vi "Lab Panel V4.90.vi"() -> ()   [LabVIEW 2013] (continued)
                            n1480 = local write "RESULT LAB05-2"(TRUE) -> ()
                            n1481 = local write "DISP LAB05-2"(w2794) -> ()
                          }
                        }
                      }
                      frame False {
                      }
                    }
                  }
                }
              }
            }
          }
          frame #6 {
            # "end test & close test files"
            n1482 = local read "MAIL SETTINGS"() -> (w2800:T7)
            n1483 = Unbundle(w2800) -> ("OUT SERVER ADDRESS"=w2799:string, "FROM ACCOUNT"=w2798:string)  [unwired: 5 out]
            n1484 = stacked-sequence {
              tunnel: w2810 -> [_ _ _ _ _ _ _ _ _ _]
              tunnel: w2811 -> [_ _ _ _ _ _ _ _ _ _]
              tunnel: w2809 -> [_ _ _ _ _ _ _ _ _ _]
              tunnel: w2808 -> [_ _ _ _ _ _ _ _ _ _]
              tunnel: w2807 -> [_ _ _ _ _ _ _ _ _ _]
              tunnel: w2806 -> [_ _ _ _ _ _ _ _ _ _]
              tunnel: w2805 -> [_ _ _ _ _ _ _ _ _ _]
              tunnel: w2804 -> [_ _ _ _ _ _ _ _ _ _]
              tunnel: w2803 -> [_ _ _ _ _ _ _ _ _ _]
              tunnel: w2802 -> [_ _ _ _ _ _ _ _ _ _]
              tunnel: w2799 -> [w2815 w2867 w2915 w2962 w3009 w3056 w3103 w3150 w3197 w3244]
              tunnel: w2798 -> [w2814 w2866 w2914 w2961 w3008 w3055 w3102 w3149 w3196 w3243]
              tunnel: "Mail Test File To:" -> [w2813 w2865 w2913 w2960 w3007 w3054 w3101 w3148 w3195 w3242]
              tunnel: "Mail Test Fail" -> [w2812 w2864 w2912 w2959 w3006 w3053 w3100 w3147 w3194 w3241]
              frame #0 {
                # "LAB01-1"
                n1485 = local read "DISP LAB01-1"() -> (w2819:T4)
                n1486 = local read "run lab01-1"() -> (w2816:bool)
                n1487 = local read "TDMS LAB01-1"() -> (w2817:refnum<k34>)
                n1488 = Unbundle(w2819) -> ("CYCLE"=w2820:dbl, "STATUS"=w2818:string)  [unwired: 1 out]
                n1489 = case shown="True" w2816 {
                  tunnel: w2820 -> [_ w2826]
                  tunnel: w2819 -> [_ w2828]
                  tunnel: w2818 -> [_ w2825]
                  tunnel: w2817 -> [_ w2827]
                  tunnel: w2815 -> [_ w2824]
                  tunnel: w2814 -> [_ w2823]
                  tunnel: w2813 -> [_ w2822]
                  tunnel: w2812 -> [_ w2821]
                  frame False {
                  }
                  frame True {
                    n1490 = Not Equal?(x=w2825, y="RUN") -> (x != y?=w2829:bool)
                    n1491 = Greater?(x=w2826, y=2.0) -> (0:w2831:bool)
                    n1492 = And(x=w2831, y=w2829) -> (x .and. y?=w2830:bool)
                    n1493 = case shown="True" w2830 {
                      tunnel: w2828 -> [_ w2841]
                      tunnel: w2827 -> [_ w2840]
                      tunnel: w2826 -> [_ w2839]
                      tunnel: w2825 -> [_ w2838]
                      tunnel: w2824 -> [_ w2837]
                      tunnel: w2823 -> [_ w2836]
                      tunnel: w2822 -> [_ w2835]
                      tunnel: w2821 -> [_ w2834]
                      frame False {
                      }
                      frame True {
                        n1494 = stacked-sequence {
                          tunnel: w2841 -> [w2845 _ _]
                          tunnel: w2840 -> [_ w2847 _]
                          tunnel: w2839 -> [_ _ _]
                          tunnel: w2838 -> [_ _ w2853]
                          tunnel: w2837 -> [_ _ w2852]
                          tunnel: w2836 -> [_ _ w2851]
                          tunnel: w2835 -> [_ _ w2850]
                          tunnel: w2834 -> [_ _ w2849]
                          frame #0 {
                            w2842 = FALSE
                            n1495 = local write "mail control"("END") -> ()
                            n1496 = Bundle(cluster=w2845) -> (w2844:T4)  [unwired: 3 in]
                            n1497 = local write "DISP LAB01-1"(w2844) -> ()
                            n1498 = local write "O/I  LAB01-1"(w2842) -> ()
                            n1499 = local write "run lab01-1"(w2842) -> ()
                            n1500 = local write "RUN LAB01-1"(w2842) -> ()
                          }
                          frame #1 {
                            n1501 = TDMS Close(11:w2847) -> (0:w2846:errorcluster)  [unwired: 1 in, 1 out]
                            n1502 = local write "data file error"(w2846) -> ()
                          }
                          frame #2 {
                            n1503 = stacked-sequence {
                              tunnel: "LAB01-1" -> [w2855 w2857 _]
                              tunnel: w2853 -> [_ w2863 _]
                              tunnel: w2852 -> [_ w2862 _]
                              tunnel: w2851 -> [_ w2861 _]
                              tunnel: w2850 -> [_ w2860 _]
                              tunnel: w2849 -> [_ w2859 _]
                              frame #0 {
                                n1504 = call "sub vi - defrag tdms v1.vi"("panel id"=w2855) -> ("error out"=w2854:errorcluster)  [unwired: 10 in]
                                n1505 = local write "data file error"(w2854) -> ()
                              }
                              frame #1 {
                                n1506 = Bundle("STATUS"=w2863, "OUT SERVER ADDRESS"=w2862, "FROM ACCOUNT"=w2861, "Mail Test File To:"=w2860, "Mail Test Fail"=w2859) -> (w2856:T25)  [unwired: 1 in]
                                n1507 = call "Save data file (pass-fail) v5.vi"("Input Cluster"=w2856, "panel id"=w2857) -> ("network file save error"=w2858:errorcluster)  [unwired: 8 in, 1 out]
                                n1508 = local write "data file error"(w2858) -> ()
                              }
                              frame #2 {
                              }
                            }
                          }
                        }
                      }
                    }
                  }
                }
              }
              frame #1 {
                # "LAB01-2"
                n1509 = local read "run lab01-2"() -> (w2868:bool)
                n1510 = case shown="True" w2868 {
                  tunnel: w2867 -> [_ w2872]
                  tunnel: w2866 -> [_ w2871]
                  tunnel: w2865 -> [_ w2870]
                  tunnel: w2864 -> [_ w2869]
                  frame False {
                  }
                  frame True {
                    n1511 = local read "DISP LAB01-2"() -> (w2880:T4)
                    n1512 = local read "TDMS LAB01-2"() -> (w2879:refnum<k34>)
                    n1513 = Unbundle(w2880) -> ("CYCLE"=w2874:dbl, "STATUS"=w2873:string)  [unwired: 1 out]
                    n1514 = Not Equal?(x=w2873, y="RUN") -> (x != y?=w2876:bool)
                    n1515 = Greater?(x=w2874, y=2.0) -> (0:w2877:bool)
                    n1516 = And(x=w2877, y=w2876) -> (x .and. y?=w2875:bool)
                    n1517 = case shown="True" w2875 {
                      tunnel: w2880 -> [_ w2889]
                      tunnel: w2879 -> [_ w2888]
                      tunnel: w2874 -> [_ w2887]
                      tunnel: w2873 -> [_ w2886]
                      tunnel: w2872 -> [_ w2885]
                      tunnel: w2871 -> [_ w2884]
                      tunnel: w2870 -> [_ w2883]
                      tunnel: w2869 -> [_ w2882]
                      frame False {
                      }
                      frame True {
                        n1518 = stacked-sequence {
                          tunnel: w2889 -> [w2892 _ _]
                          tunnel: w2888 -> [_ w2894 _]
                          tunnel: w2887 -> [_ _ _]
                          tunnel: w2886 -> [_ _ w2900]
                          tunnel: w2885 -> [_ _ w2899]
                          tunnel: w2884 -> [_ _ w2898]
                          tunnel: w2883 -> [_ _ w2897]
                          tunnel: w2882 -> [_ _ w2896]
                          frame #0 {
                            w2890 = FALSE
                            n1519 = local write "mail control"("END") -> ()
                            n1520 = Bundle(cluster=w2892) -> (w2893:T4)  [unwired: 3 in]
                            n1521 = local write "RUN LAB01-2"(w2890) -> ()
                            n1522 = local write "run lab01-2"(w2890) -> ()
                            n1523 = local write "O/I  LAB01-2"(w2890) -> ()
                            n1524 = local write "DISP LAB01-2"(w2893) -> ()
                          }
                          frame #1 {
                            n1525 = TDMS Close(11:w2894) -> (0:w2895:errorcluster)  [unwired: 1 in, 1 out]
                            n1526 = local write "data file error"(w2895) -> ()
                          }
                          frame #2 {
                            n1527 = stacked-sequence {
                              tunnel: "LAB01-2" -> [w2903 w2904]
                              tunnel: w2900 -> [_ w2909]
                              tunnel: w2899 -> [_ w2908]
                              tunnel: w2898 -> [_ w2907]
                              tunnel: w2897 -> [_ w2906]
                              tunnel: w2896 -> [_ w2905]
                              frame #0 {
                                n1528 = call "sub vi - defrag tdms v1.vi"("panel id"=w2903) -> ("error out"=w2902:errorcluster)  [unwired: 10 in]
                                n1529 = local write "data file error"(w2902) -> ()
                              }
                              frame #1 {
                                n1530 = Bundle("STATUS"=w2909, "OUT SERVER ADDRESS"=w2908, "FROM ACCOUNT"=w2907, "Mail Test File To:"=w2906, "Mail Test Fail"=w2905) -> (w2911:T25)  [unwired: 1 in]
                                n1531 = call "Save data file (pass-fail) v5.vi"("Input Cluster"=w2911, "panel id"=w2904) -> ("network file save error"=w2910:errorcluster)  [unwired: 8 in, 1 out]
                                n1532 = local write "data file error"(w2910) -> ()
                              }
                            }
                          }
                        }
                      }
                    }
                  }
                }
              }
              frame #2 {
                # "LAB02-1"
                n1533 = local read "run lab02-1"() -> (w2916:bool)
                n1534 = case shown="True" w2916 {
                  tunnel: w2915 -> [_ w2920]
                  tunnel: w2914 -> [_ w2919]
                  tunnel: w2913 -> [_ w2918]
                  tunnel: w2912 -> [_ w2917]
                  frame False {
                  }
                  frame True {
                    n1535 = local read "DISP LAB02-1"() -> (w2928:T4)
                    n1536 = Unbundle(w2928) -> ("CYCLE"=w2924:dbl, "STATUS"=w2921:string)  [unwired: 1 out]
                    n1537 = local read "TDMS LAB02-1"() -> (w2927:refnum<k34>)
                    n1538 = Not Equal?(x=w2921, y="RUN") -> (x != y?=w2923:bool)
                    n1539 = Greater?(x=w2924, y=2.0) -> (0:w2925:bool)
                    n1540 = And(x=w2925, y=w2923) -> (x .and. y?=w2922:bool)
                    n1541 = case shown="True" w2922 {
                      tunnel: w2928 -> [_ w2936]
                      tunnel: w2927 -> [_ w2935]
                      tunnel: w2921 -> [_ w2934]
                      tunnel: w2920 -> [_ w2933]
                      tunnel: w2919 -> [_ w2932]
                      tunnel: w2918 -> [_ w2931]
                      tunnel: w2917 -> [_ w2930]
                      frame False {
                      }
                      frame True {
                        n1542 = stacked-sequence {
                          tunnel: w2936 -> [w2939 _ _]
                          tunnel: w2935 -> [_ w2941 _]
                          tunnel: w2934 -> [_ _ w2947]
                          tunnel: w2933 -> [_ _ w2946]
                          tunnel: w2932 -> [_ _ w2945]
                          tunnel: w2931 -> [_ _ w2944]
                          tunnel: w2930 -> [_ _ w2943]
                          frame #0 {
                            w2937 = FALSE
                            n1543 = local write "mail control"("END") -> ()
                            n1544 = Bundle(cluster=w2939) -> (w2940:T4)  [unwired: 3 in]
                            n1545 = local write "O/I  LAB02-1"(w2937) -> ()
                            n1546 = local write "RUN LAB02-1"(w2937) -> ()
                            n1547 = local write "run lab02-1"(w2937) -> ()
                            n1548 = local write "DISP LAB02-1"(w2940) -> ()
                          }
                          frame #1 {
                            n1549 = TDMS Close(11:w2941) -> (0:w2942:errorcluster)  [unwired: 1 in, 1 out]
                            n1550 = local write "data file error"(w2942) -> ()
                          }
                          frame #2 {
                            n1551 = stacked-sequence {
                              tunnel: "LAB02-1" -> [w2950 w2957]
                              tunnel: w2947 -> [_ w2955]
                              tunnel: w2946 -> [_ w2954]
                              tunnel: w2945 -> [_ w2953]
                              tunnel: w2944 -> [_ w2952]
                              tunnel: w2943 -> [_ w2951]
                              frame #0 {
                                n1552 = call "sub vi - defrag tdms v1.vi"("panel id"=w2950) -> ("error out"=w2949:errorcluster)  [unwired: 10 in]
                                n1553 = local write "data file error"(w2949) -> ()
                              }
                              frame #1 {
                                n1554 = Bundle("STATUS"=w2955, "OUT SERVER ADDRESS"=w2954, "FROM ACCOUNT"=w2953, "Mail Test File To:"=w2952, "Mail Test Fail"=w2951) -> (w2956:T25)  [unwired: 1 in]
                                n1555 = call "Save data file (pass-fail) v5.vi"("Input Cluster"=w2956, "panel id"=w2957) -> ("network file save error"=w2958:errorcluster)  [unwired: 8 in, 1 out]
                                n1556 = local write "data file error"(w2958) -> ()
                              }
                            }
                          }
                        }
                      }
                    }
                  }
                }
              }
              frame #3 {
                # "LAB02-2"
                n1557 = local read "run lab02-2"() -> (w2963:bool)
                n1558 = case shown="True" w2963 {
                  tunnel: w2962 -> [_ w2967]
                  tunnel: w2961 -> [_ w2966]
                  tunnel: w2960 -> [_ w2965]
                  tunnel: w2959 -> [_ w2964]
                  frame False {
                  }
                  frame True {
                    n1559 = local read "DISP LAB02-2"() -> (w2975:T4)
                    n1560 = local read "TDMS LAB02-2"() -> (w2974:refnum<k34>)
                    n1561 = Unbundle(w2975) -> ("CYCLE"=w2971:dbl, "STATUS"=w2968:string)  [unwired: 1 out]
                    n1562 = Not Equal?(x=w2968, y="RUN") -> (x != y?=w2970:bool)
                    n1563 = Greater?(x=w2971, y=2.0) -> (0:w2972:bool)
                    n1564 = And(x=w2972, y=w2970) -> (x .and. y?=w2969:bool)
                    n1565 = case shown="True" w2969 {
                      tunnel: w2975 -> [_ w2983]
                      tunnel: w2974 -> [_ w2982]
                      tunnel: w2968 -> [_ w2981]
                      tunnel: w2967 -> [_ w2980]
                      tunnel: w2966 -> [_ w2979]
                      tunnel: w2965 -> [_ w2978]
                      tunnel: w2964 -> [_ w2977]
                      frame False {
                      }
                      frame True {
                        n1566 = stacked-sequence {
                          tunnel: w2983 -> [w2986 _ _]
                          tunnel: w2982 -> [_ w2988 _]
                          tunnel: w2981 -> [_ _ w2994]
                          tunnel: w2980 -> [_ _ w2993]
                          tunnel: w2979 -> [_ _ w2992]
                          tunnel: w2978 -> [_ _ w2991]
                          tunnel: w2977 -> [_ _ w2990]
                          frame #0 {
                            w2984 = FALSE
                            n1567 = local write "mail control"("END") -> ()
                            n1568 = Bundle(cluster=w2986) -> (w2987:T4)  [unwired: 3 in]
                            n1569 = local write "O/I  LAB02-2"(w2984) -> ()
                            n1570 = local write "run lab02-2"(w2984) -> ()
                            n1571 = local write "RUN LAB02-2"(w2984) -> ()
                            n1572 = local write "DISP LAB02-2"(w2987) -> ()
                          }
                          frame #1 {
                            n1573 = TDMS Close(11:w2988) -> (0:w2989:errorcluster)  [unwired: 1 in, 1 out]
                            n1574 = local write "data file error"(w2989) -> ()
                          }
                          frame #2 {
                            n1575 = stacked-sequence {
                              tunnel: "LAB02-2" -> [w2997 w3003]
                              tunnel: w2994 -> [_ w3002]
                              tunnel: w2993 -> [_ w3001]
                              tunnel: w2992 -> [_ w3000]
                              tunnel: w2991 -> [_ w2999]
                              tunnel: w2990 -> [_ w2998]
                              frame #0 {
                                n1576 = call "sub vi - defrag tdms v1.vi"("panel id"=w2997) -> ("error out"=w2996:errorcluster)  [unwired: 10 in]
                                n1577 = local write "data file error"(w2996) -> ()
                              }
                              frame #1 {
                                n1578 = Bundle("STATUS"=w3002, "OUT SERVER ADDRESS"=w3001, "FROM ACCOUNT"=w3000, "Mail Test File To:"=w2999, "Mail Test Fail"=w2998) -> (w3005:T25)  [unwired: 1 in]
                                n1579 = call "Save data file (pass-fail) v5.vi"("Input Cluster"=w3005, "panel id"=w3003) -> ("network file save error"=w3004:errorcluster)  [unwired: 8 in, 1 out]
                                n1580 = local write "data file error"(w3004) -> ()
                              }
                            }
                          }
                        }
                      }
                    }
                  }
                }
              }
              frame #4 {
                # "LAB03-1"
                n1581 = local read "run lab03-1"() -> (w3010:bool)
                n1582 = case shown="True" w3010 {
                  tunnel: w3009 -> [_ w3014]
                  tunnel: w3008 -> [_ w3013]
                  tunnel: w3007 -> [_ w3012]
                  tunnel: w3006 -> [_ w3011]
                  frame False {
                  }
                  frame True {
                    n1583 = local read "DISP LAB03-1"() -> (w3022:T4)
                    n1584 = local read "TDMS LAB03-1"() -> (w3021:refnum<k34>)
                    n1585 = Unbundle(w3022) -> ("CYCLE"=w3018:dbl, "STATUS"=w3015:string)  [unwired: 1 out]
                    n1586 = Not Equal?(x=w3015, y="RUN") -> (x != y?=w3017:bool)
                    n1587 = Greater?(x=w3018, y=2.0) -> (0:w3019:bool)
                    n1588 = And(x=w3019, y=w3017) -> (x .and. y?=w3016:bool)
                    n1589 = case shown="True" w3016 {
                      tunnel: w3022 -> [_ w3030]
                      tunnel: w3021 -> [_ w3029]
                      tunnel: w3015 -> [_ w3028]
                      tunnel: w3014 -> [_ w3027]
                      tunnel: w3013 -> [_ w3026]
                      tunnel: w3012 -> [_ w3025]
                      tunnel: w3011 -> [_ w3024]
                      frame False {
                      }
                      frame True {
                        n1590 = stacked-sequence {
                          tunnel: w3030 -> [w3033 _ _]
                          tunnel: w3029 -> [_ w3035 _]
                          tunnel: w3028 -> [_ _ w3041]
                          tunnel: w3027 -> [_ _ w3040]
                          tunnel: w3026 -> [_ _ w3039]
                          tunnel: w3025 -> [_ _ w3038]
                          tunnel: w3024 -> [_ _ w3037]
                          frame #0 {
                            w3031 = FALSE
                            n1591 = local write "mail control"("END") -> ()
                            n1592 = Bundle(cluster=w3033) -> (w3034:T4)  [unwired: 3 in]
                            n1593 = local write "O/I  LAB03-1"(w3031) -> ()
                            n1594 = local write "run lab03-1"(w3031) -> ()
                            n1595 = local write "RUN LAB03-1"(w3031) -> ()
                            n1596 = local write "DISP LAB03-1"(w3034) -> ()
                          }
                          frame #1 {
                            n1597 = TDMS Close(11:w3035) -> (0:w3036:errorcluster)  [unwired: 1 in, 1 out]
                            n1598 = local write "data file error"(w3036) -> ()
                          }
                          frame #2 {
                            n1599 = stacked-sequence {
                              tunnel: "LAB03-1" -> [w3044 w3050]
                              tunnel: w3041 -> [_ w3049]
                              tunnel: w3040 -> [_ w3048]
                              tunnel: w3039 -> [_ w3047]
                              tunnel: w3038 -> [_ w3046]
                              tunnel: w3037 -> [_ w3045]
                              frame #0 {
                                n1600 = call "sub vi - defrag tdms v1.vi"("panel id"=w3044) -> ("error out"=w3043:errorcluster)  [unwired: 10 in]
                                n1601 = local write "data file error"(w3043) -> ()
                              }
                              frame #1 {
                                n1602 = Bundle("STATUS"=w3049, "OUT SERVER ADDRESS"=w3048, "FROM ACCOUNT"=w3047, "Mail Test File To:"=w3046, "Mail Test Fail"=w3045) -> (w3052:T25)  [unwired: 1 in]
                                n1603 = call "Save data file (pass-fail) v5.vi"("Input Cluster"=w3052, "panel id"=w3050) -> ("network file save error"=w3051:errorcluster)  [unwired: 8 in, 1 out]
                                n1604 = local write "data file error"(w3051) -> ()
                              }
                            }
                          }
                        }
                      }
                    }
                  }
                }
              }
              frame #5 {
                # "LAB03-2"
                n1605 = local read "run lab03-2"() -> (w3057:bool)
                n1606 = case shown="True" w3057 {
                  tunnel: w3056 -> [_ w3061]
                  tunnel: w3055 -> [_ w3060]
                  tunnel: w3054 -> [_ w3059]
                  tunnel: w3053 -> [_ w3058]
                  frame False {
                  }
                  frame True {
                    n1607 = local read "DISP LAB03-2"() -> (w3069:T4)
                    n1608 = Unbundle(w3069) -> ("CYCLE"=w3065:dbl, "STATUS"=w3062:string)  [unwired: 1 out]
                    n1609 = local read "TDMS LAB03-2"() -> (w3068:refnum<k34>)
                    n1610 = Not Equal?(x=w3062, y="RUN") -> (x != y?=w3064:bool)
                    n1611 = Greater?(x=w3065, y=2.0) -> (0:w3066:bool)
                    n1612 = And(x=w3066, y=w3064) -> (x .and. y?=w3063:bool)
                    n1613 = case shown="True" w3063 {
                      tunnel: w3069 -> [_ w3077]
                      tunnel: w3068 -> [_ w3076]
                      tunnel: w3062 -> [_ w3075]
                      tunnel: w3061 -> [_ w3074]
                      tunnel: w3060 -> [_ w3073]
                      tunnel: w3059 -> [_ w3072]
                      tunnel: w3058 -> [_ w3071]
                      frame False {
                      }
                      frame True {
                        n1614 = stacked-sequence {
                          tunnel: w3077 -> [w3080 _ _]
                          tunnel: w3076 -> [_ w3082 _]
                          tunnel: w3075 -> [_ _ w3088]
                          tunnel: w3074 -> [_ _ w3087]
                          tunnel: w3073 -> [_ _ w3086]
                          tunnel: w3072 -> [_ _ w3085]
                          tunnel: w3071 -> [_ _ w3084]
                          frame #0 {
                            w3078 = FALSE
                            n1615 = local write "mail control"("END") -> ()
                            n1616 = Bundle(cluster=w3080) -> (w3081:T4)  [unwired: 3 in]
                            n1617 = local write "RUN LAB03-2"(w3078) -> ()
                            n1618 = local write "O/I  LAB03-2"(w3078) -> ()
                            n1619 = local write "DISP LAB03-2"(w3081) -> ()
                            n1620 = local write "run lab03-2"(w3078) -> ()
                          }
                          frame #1 {
                            n1621 = TDMS Close(11:w3082) -> (0:w3083:errorcluster)  [unwired: 1 in, 1 out]
                            n1622 = local write "data file error"(w3083) -> ()
                          }
                          frame #2 {
                            n1623 = stacked-sequence {
                              tunnel: "LAB03-2" -> [w3091 w3092]
                              tunnel: w3088 -> [_ w3097]
                              tunnel: w3087 -> [_ w3096]
                              tunnel: w3086 -> [_ w3095]
                              tunnel: w3085 -> [_ w3094]
                              tunnel: w3084 -> [_ w3093]
                              frame #0 {
                                n1624 = call "sub vi - defrag tdms v1.vi"("panel id"=w3091) -> ("error out"=w3090:errorcluster)  [unwired: 10 in]
                                n1625 = local write "data file error"(w3090) -> ()
                              }
                              frame #1 {
                                n1626 = Bundle("STATUS"=w3097, "OUT SERVER ADDRESS"=w3096, "FROM ACCOUNT"=w3095, "Mail Test File To:"=w3094, "Mail Test Fail"=w3093) -> (w3099:T25)  [unwired: 1 in]
                                n1627 = call "Save data file (pass-fail) v5.vi"("Input Cluster"=w3099, "panel id"=w3092) -> ("network file save error"=w3098:errorcluster)  [unwired: 8 in, 1 out]
                                n1628 = local write "data file error"(w3098) -> ()
                              }
                            }
                          }
                        }
                      }
                    }
                  }
                }
              }
              frame #6 {
                # "LAB04-1"
                n1629 = local read "run lab04-1"() -> (w3104:bool)
                n1630 = case shown="True" w3104 {
                  tunnel: w3103 -> [_ w3108]
                  tunnel: w3102 -> [_ w3107]
                  tunnel: w3101 -> [_ w3106]
                  tunnel: w3100 -> [_ w3105]
                  frame False {
                  }
                  frame True {
                    n1631 = local read "DISP LAB04-1"() -> (w3116:T4)
                    n1632 = Unbundle(w3116) -> ("CYCLE"=w3112:dbl, "STATUS"=w3109:string)  [unwired: 1 out]
                    n1633 = local read "TDMS LAB04-1"() -> (w3115:refnum<k34>)
                    n1634 = Not Equal?(x=w3109, y="RUN") -> (x != y?=w3111:bool)
                    n1635 = Greater?(x=w3112, y=2.0) -> (0:w3113:bool)
                    n1636 = And(x=w3113, y=w3111) -> (x .and. y?=w3110:bool)
                    n1637 = case shown="True" w3110 {
                      tunnel: w3116 -> [_ w3124]
                      tunnel: w3115 -> [_ w3123]
                      tunnel: w3109 -> [_ w3122]
                      tunnel: w3108 -> [_ w3121]
                      tunnel: w3107 -> [_ w3120]
                      tunnel: w3106 -> [_ w3119]
                      tunnel: w3105 -> [_ w3118]
                      frame False {
                      }
                      frame True {
                        n1638 = stacked-sequence {
                          tunnel: w3124 -> [w3127 _ _]
                          tunnel: w3123 -> [_ w3129 _]
                          tunnel: w3122 -> [_ _ w3135]
                          tunnel: w3121 -> [_ _ w3134]
                          tunnel: w3120 -> [_ _ w3133]
                          tunnel: w3119 -> [_ _ w3132]
                          tunnel: w3118 -> [_ _ w3131]
                          frame #0 {
                            w3125 = FALSE
                            n1639 = local write "mail control"("END") -> ()
                            n1640 = Bundle(cluster=w3127) -> (w3128:T4)  [unwired: 3 in]
                            n1641 = local write "RUN LAB04-1"(w3125) -> ()
                            n1642 = local write "O/I  LAB04-1"(w3125) -> ()
                            n1643 = local write "run lab04-1"(w3125) -> ()
                            n1644 = local write "DISP LAB04-1"(w3128) -> ()
                          }
                          frame #1 {
                            n1645 = TDMS Close(11:w3129) -> (0:w3130:errorcluster)  [unwired: 1 in, 1 out]
                            n1646 = local write "data file error"(w3130) -> ()
                          }
                          frame #2 {
                            n1647 = stacked-sequence {
                              tunnel: "LAB04-1" -> [w3138 w3139]
                              tunnel: w3135 -> [_ w3144]
                              tunnel: w3134 -> [_ w3143]
                              tunnel: w3133 -> [_ w3142]
                              tunnel: w3132 -> [_ w3141]
                              tunnel: w3131 -> [_ w3140]
                              frame #0 {
                                n1648 = call "sub vi - defrag tdms v1.vi"("panel id"=w3138) -> ("error out"=w3137:errorcluster)  [unwired: 10 in]
                                n1649 = local write "data file error"(w3137) -> ()
                              }
                              frame #1 {
                                n1650 = Bundle("STATUS"=w3144, "OUT SERVER ADDRESS"=w3143, "FROM ACCOUNT"=w3142, "Mail Test File To:"=w3141, "Mail Test Fail"=w3140) -> (w3146:T25)  [unwired: 1 in]
                                n1651 = call "Save data file (pass-fail) v5.vi"("Input Cluster"=w3146, "panel id"=w3139) -> ("network file save error"=w3145:errorcluster)  [unwired: 8 in, 1 out]
                                n1652 = local write "data file error"(w3145) -> ()
                              }
                            }
                          }
                        }
                      }
                    }
                  }
                }
              }
              frame #7 {
                # "LAB04-2"
                n1653 = local read "run lab04-2"() -> (w3151:bool)
                n1654 = case shown="True" w3151 {
                  tunnel: w3150 -> [_ w3155]
                  tunnel: w3149 -> [_ w3154]
                  tunnel: w3148 -> [_ w3153]
                  tunnel: w3147 -> [_ w3152]
                  frame False {
                  }
                  frame True {
                    n1655 = local read "DISP LAB04-2"() -> (w3163:T4)
                    n1656 = Unbundle(w3163) -> ("CYCLE"=w3159:dbl, "STATUS"=w3156:string)  [unwired: 1 out]
                    n1657 = Not Equal?(x=w3156, y="RUN") -> (x != y?=w3158:bool)
                    n1658 = local read "TDMS LAB04-2"() -> (w3162:refnum<k34>)
                    n1659 = Greater?(x=w3159, y=2.0) -> (0:w3160:bool)
                    n1660 = And(x=w3160, y=w3158) -> (x .and. y?=w3157:bool)
                    n1661 = case shown="True" w3157 {
                      tunnel: w3163 -> [_ w3171]
                      tunnel: w3162 -> [_ w3170]
                      tunnel: w3156 -> [_ w3169]
                      tunnel: w3155 -> [_ w3168]
                      tunnel: w3154 -> [_ w3167]
                      tunnel: w3153 -> [_ w3166]
                      tunnel: w3152 -> [_ w3165]
                      frame False {
                      }
                      frame True {
                        n1662 = stacked-sequence {
                          tunnel: w3171 -> [w3174 _ _]
                          tunnel: w3170 -> [_ w3176 _]
                          tunnel: w3169 -> [_ _ w3182]
                          tunnel: w3168 -> [_ _ w3181]
                          tunnel: w3167 -> [_ _ w3180]
                          tunnel: w3166 -> [_ _ w3179]
                          tunnel: w3165 -> [_ _ w3178]
                          frame #0 {
                            w3172 = FALSE
                            n1663 = local write "mail control"("END") -> ()
                            n1664 = Bundle(cluster=w3174) -> (w3175:T4)  [unwired: 3 in]
                            n1665 = local write "O/I  LAB04-2"(w3172) -> ()
                            n1666 = local write "RUN LAB04-2"(w3172) -> ()
                            n1667 = local write "run lab04-2"(w3172) -> ()
                            n1668 = local write "DISP LAB04-2"(w3175) -> ()
                          }
                          frame #1 {
                            n1669 = TDMS Close(11:w3176) -> (0:w3177:errorcluster)  [unwired: 1 in, 1 out]
                            n1670 = local write "data file error"(w3177) -> ()
                          }
                          frame #2 {
                            n1671 = stacked-sequence {
                              tunnel: "LAB04-2" -> [w3185 w3186]
                              tunnel: w3182 -> [_ w3191]
                              tunnel: w3181 -> [_ w3190]
                              tunnel: w3180 -> [_ w3189]
                              tunnel: w3179 -> [_ w3188]
                              tunnel: w3178 -> [_ w3187]
                              frame #0 {
                                n1672 = call "sub vi - defrag tdms v1.vi"("panel id"=w3185) -> ("error out"=w3184:errorcluster)  [unwired: 10 in]
                                n1673 = local write "data file error"(w3184) -> ()
                              }
                              frame #1 {
                                n1674 = Bundle("STATUS"=w3191, "OUT SERVER ADDRESS"=w3190, "FROM ACCOUNT"=w3189, "Mail Test File To:"=w3188, "Mail Test Fail"=w3187) -> (w3193:T25)  [unwired: 1 in]
                                n1675 = call "Save data file (pass-fail) v5.vi"("Input Cluster"=w3193, "panel id"=w3186) -> ("network file save error"=w3192:errorcluster)  [unwired: 8 in, 1 out]
                                n1676 = local write "data file error"(w3192) -> ()
                              }
                            }
                          }
                        }
                      }
                    }
                  }
                }
              }
              frame #8 {
                # "LAB05-1"
                n1677 = local read "run lab05-1"() -> (w3198:bool)
                n1678 = case shown="True" w3198 {
                  tunnel: w3197 -> [_ w3202]
                  tunnel: w3196 -> [_ w3201]
                  tunnel: w3195 -> [_ w3200]
                  tunnel: w3194 -> [_ w3199]
                  frame False {
                  }
                  frame True {
                    n1679 = local read "DISP LAB05-1"() -> (w3210:T4)
                    n1680 = Unbundle(w3210) -> ("CYCLE"=w3206:dbl, "STATUS"=w3203:string)  [unwired: 1 out]
                    n1681 = Not Equal?(x=w3203, y="RUN") -> (x != y?=w3205:bool)
                    n1682 = local read "TDMS LAB05-1"() -> (w3209:refnum<k34>)
                    n1683 = Greater?(x=w3206, y=2.0) -> (0:w3207:bool)
                    n1684 = And(x=w3207, y=w3205) -> (x .and. y?=w3204:bool)
                    n1685 = case shown="True" w3204 {
                      tunnel: w3210 -> [_ w3218]
                      tunnel: w3209 -> [_ w3217]
                      tunnel: w3203 -> [_ w3216]
                      tunnel: w3202 -> [_ w3215]
                      tunnel: w3201 -> [_ w3214]
                      tunnel: w3200 -> [_ w3213]
                      tunnel: w3199 -> [_ w3212]
                      frame False {
                      }
                      frame True {
                        n1686 = stacked-sequence {
                          tunnel: w3218 -> [w3221 _ _]
                          tunnel: w3217 -> [_ w3223 _]
                          tunnel: w3216 -> [_ _ w3229]
                          tunnel: w3215 -> [_ _ w3228]
                          tunnel: w3214 -> [_ _ w3227]
                          tunnel: w3213 -> [_ _ w3226]
                          tunnel: w3212 -> [_ _ w3225]
                          frame #0 {
                            w3219 = FALSE
                            n1687 = local write "mail control"("END") -> ()
                            n1688 = Bundle(cluster=w3221) -> (w3222:T4)  [unwired: 3 in]
                            n1689 = local write "O/I  LAB05-1"(w3219) -> ()
                            n1690 = local write "RUN LAB05-1"(w3219) -> ()
                            n1691 = local write "run lab05-1"(w3219) -> ()
                            n1692 = local write "DISP LAB05-1"(w3222) -> ()
                          }
                          frame #1 {
                            n1693 = TDMS Close(11:w3223) -> (0:w3224:errorcluster)  [unwired: 1 in, 1 out]
                            n1694 = local write "data file error"(w3224) -> ()
                          }
                          frame #2 {
                            n1695 = stacked-sequence {
                              tunnel: "LAB05-1" -> [w3232 w3238]
                              tunnel: w3229 -> [_ w3237]
                              tunnel: w3228 -> [_ w3236]
                              tunnel: w3227 -> [_ w3235]
                              tunnel: w3226 -> [_ w3234]
                              tunnel: w3225 -> [_ w3233]
                              frame #0 {
                                n1696 = call "sub vi - defrag tdms v1.vi"("panel id"=w3232) -> ("error out"=w3231:errorcluster)  [unwired: 10 in]
                                n1697 = local write "data file error"(w3231) -> ()
                              }
                              frame #1 {
                                n1698 = Bundle("STATUS"=w3237, "OUT SERVER ADDRESS"=w3236, "FROM ACCOUNT"=w3235, "Mail Test File To:"=w3234, "Mail Test Fail"=w3233) -> (w3240:T25)  [unwired: 1 in]
                                n1699 = call "Save data file (pass-fail) v5.vi"("Input Cluster"=w3240, "panel id"=w3238) -> ("network file save error"=w3239:errorcluster)  [unwired: 8 in, 1 out]
                                n1700 = local write "data file error"(w3239) -> ()
                              }
                            }
                          }
                        }
                      }
                    }
                  }
                }
              }
              frame #9 {
                # "LAB05-2"
                n1701 = local read "run lab05-2"() -> (w3245:bool)
                n1702 = case shown="True" w3245 {
                  tunnel: w3244 -> [_ w3249]
                  tunnel: w3243 -> [_ w3248]
                  tunnel: w3242 -> [_ w3247]
                  tunnel: w3241 -> [_ w3246]
                  frame False {
                  }
                  frame True {
                    n1703 = local read "DISP LAB05-2"() -> (w3257:T4)
                    n1704 = Unbundle(w3257) -> ("CYCLE"=w3253:dbl, "STATUS"=w3250:string)  [unwired: 1 out]
                    n1705 = Not Equal?(x=w3250, y="RUN") -> (x != y?=w3252:bool)
                    n1706 = local read "TDMS LAB05-2"() -> (w3256:refnum<k34>)
                    n1707 = Greater?(x=w3253, y=2.0) -> (0:w3254:bool)
                    n1708 = And(x=w3254, y=w3252) -> (x .and. y?=w3251:bool)
                    n1709 = case shown="True" w3251 {
                      tunnel: w3257 -> [_ w3265]
                      tunnel: w3256 -> [_ w3264]
                      tunnel: w3250 -> [_ w3263]
                      tunnel: w3249 -> [_ w3262]
                      tunnel: w3248 -> [_ w3261]
                      tunnel: w3247 -> [_ w3260]
                      tunnel: w3246 -> [_ w3259]
                      frame False {
                      }
                      frame True {
                        n1710 = stacked-sequence {
                          tunnel: w3265 -> [w3268 _ _]
                          tunnel: w3264 -> [_ w3270 _]
                          tunnel: w3263 -> [_ _ w3276]
                          tunnel: w3262 -> [_ _ w3275]
                          tunnel: w3261 -> [_ _ w3274]
                          tunnel: w3260 -> [_ _ w3273]
                          tunnel: w3259 -> [_ _ w3272]
                          frame #0 {
                            w3266 = FALSE
                            n1711 = local write "mail control"("END") -> ()
                            n1712 = Bundle(cluster=w3268) -> (w3269:T4)  [unwired: 3 in]
                            n1713 = local write "RUN LAB05-2"(w3266) -> ()
                            n1714 = local write "O/I  LAB05-2"(w3266) -> ()
                            n1715 = local write "run lab05-2"(w3266) -> ()
                            n1716 = local write "DISP LAB05-2"(w3269) -> ()
                          }
                          frame #1 {
                            n1717 = TDMS Close(11:w3270) -> (0:w3271:errorcluster)  [unwired: 1 in, 1 out]
                            n1718 = local write "data file error"(w3271) -> ()
                          }
                          frame #2 {
                            n1719 = stacked-sequence {
                              tunnel: "LAB05-2" -> [w3279 w3285]
                              tunnel: w3276 -> [_ w3284]
                              tunnel: w3275 -> [_ w3283]
                              tunnel: w3274 -> [_ w3282]
                              tunnel: w3273 -> [_ w3281]
                              tunnel: w3272 -> [_ w3280]
                              frame #0 {
                                n1720 = call "sub vi - defrag tdms v1.vi"("panel id"=w3279) -> ("error out"=w3278:errorcluster)  [unwired: 10 in]
                                n1721 = local write "data file error"(w3278) -> ()
                              }
                              frame #1 {
                                n1722 = Bundle("STATUS"=w3284, "OUT SERVER ADDRESS"=w3283, "FROM ACCOUNT"=w3282, "Mail Test File To:"=w3281, "Mail Test Fail"=w3280) -> (w3287:T25)  [unwired: 1 in]
                                n1723 = call "Save data file (pass-fail) v5.vi"("Input Cluster"=w3287, "panel id"=w3285) -> ("network file save error"=w3286:errorcluster)  [unwired: 8 in, 1 out]
                                n1724 = local write "data file error"(w3286) -> ()
                              }
                            }
                          }
                        }
                      }
                    }
                  }
                }
              }
            }
            n1725 = local read "Network Directory"() -> (w2801:path)
            n1726 = global write "Global 1.vi" "Network Drive"(w2801) -> ()
          }
          frame #7 {
            # "disable functions"
            n1727 = stacked-sequence {
              tunnel: w3297 -> [w3311 _ w3368]
              tunnel: w3296 -> [w3306 _ w3367]
              tunnel: w3295 -> [w3305 _ w3366]
              tunnel: w3294 -> [w3303 _ w3365]
              tunnel: w3293 -> [w3304 _ w3364]
              tunnel: w3292 -> [_ w3328 w3363]
              tunnel: w3291 -> [_ w3329 w3362]
              tunnel: w3290 -> [_ w3330 w3361]
              tunnel: w3289 -> [_ w3331 w3360]
              tunnel: w3288 -> [_ w3332 w3359]
              frame #0 {
                n1728 = Select(t=2, s=w3303, f=0) -> (s? t:f=w3299:i32)
                n1729 = Select(t=2, s=w3305, f=0) -> (s? t:f=w3300:i32)
                n1730 = Select(t=2, s=w3304, f=0) -> (s? t:f=w3298:i32)
                n1731 = Select(t=2, s=w3311, f=0) -> (s? t:f=w3302:i32)
                n1732 = Select(t=2, s=w3306, f=0) -> (s? t:f=w3301:i32)
                n1733 = property on="SELECT LAB02-2" class="RadioBtnsControl (strict)"("DisabledEnum"=w3299) -> ()  [unwired: 2 in, 2 out]
                n1734 = property on="SELECT LAB02-1" class="RadioBtnsControl (strict)"("DisabledEnum"=w3300) -> ()  [unwired: 2 in, 2 out]
                n1735 = property on="SELECT LAB03-1" class="RadioBtnsControl (strict)"("DisabledEnum"=w3298) -> ()  [unwired: 2 in, 2 out]
                n1736 = property on="SELECT LAB01-1" class="RadioBtnsControl (strict)"("DisabledEnum"=w3302) -> ()  [unwired: 2 in, 2 out]
                n1737 = property on="SELECT LAB01-2" class="RadioBtnsControl (strict)"("DisabledEnum"=w3301) -> ()  [unwired: 2 in, 2 out]
                n1738 = Not(x=w3311) -> (.not. x?=w3312:bool)
                n1739 = property on="RESULT LAB01-1" class="Bool (strict)"("Visible"=w3312) -> ()  [unwired: 2 in, 2 out]
                n1740 = Not(x=w3306) -> (.not. x?=w3310:bool)
                n1741 = Not(x=w3305) -> (.not. x?=w3309:bool)
                n1742 = Not(x=w3303) -> (.not. x?=w3308:bool)
                n1743 = property on="RESULT LAB01-2" class="Bool (strict)"("Visible"=w3310) -> ()  [unwired: 2 in, 2 out]
                n1744 = Not(x=w3304) -> (.not. x?=w3307:bool)
                n1745 = property on="RESULT LAB02-1" class="Bool (strict)"("Visible"=w3309) -> ()  [unwired: 2 in, 2 out]
                n1746 = property on="RESULT LAB02-2" class="Bool (strict)"("Visible"=w3308) -> ()  [unwired: 2 in, 2 out]
                n1747 = property on="RESULT LAB03-1" class="Bool (strict)"("Visible"=w3307) -> ()  [unwired: 2 in, 2 out]
                n1748 = property on="SET LAB01-1" class="Clust (strict)"("DisabledEnum"=w3302) -> ()  [unwired: 2 in, 2 out]
                n1749 = property on="SET LAB01-2" class="Clust (strict)"("DisabledEnum"=w3301) -> ()  [unwired: 2 in, 2 out]
                n1750 = property on="SET LAB02-1" class="Clust (strict)"("DisabledEnum"=w3300) -> ()  [unwired: 2 in, 2 out]
                n1751 = property on="SET LAB02-2" class="Clust (strict)"("DisabledEnum"=w3299) -> ()  [unwired: 2 in, 2 out]
                n1752 = property on="SET LAB03-1" class="Clust (strict)"("DisabledEnum"=w3298) -> ()  [unwired: 2 in, 2 out]
                n1753 = property on="O/I  LAB01-1" class="Bool (strict)"("DisabledEnum"=w3302) -> ()  [unwired: 2 in, 2 out]
                n1754 = property on="O/I  LAB01-2" class="Bool (strict)"("DisabledEnum"=w3301) -> ()  [unwired: 2 in, 2 out]
                n1755 = property on="O/I  LAB02-1" class="Bool (strict)"("DisabledEnum"=w3300) -> ()  [unwired: 2 in, 2 out]
                n1756 = property on="O/I  LAB02-2" class="Bool (strict)"("DisabledEnum"=w3299) -> ()  [unwired: 2 in, 2 out]
                n1757 = property on="O/I  LAB03-1" class="Bool (strict)"("DisabledEnum"=w3298) -> ()  [unwired: 2 in, 2 out]
              }
              frame #1 {
                n1758 = Select(t=2, s=w3332, f=0) -> (s? t:f=w3323:i32)
                n1759 = Select(t=2, s=w3331, f=0) -> (s? t:f=w3324:i32)
                n1760 = Select(t=2, s=w3328, f=0) -> (s? t:f=w3327:i32)
                n1761 = Select(t=2, s=w3329, f=0) -> (s? t:f=w3326:i32)
                n1762 = Select(t=2, s=w3330, f=0) -> (s? t:f=w3325:i32)
                n1763 = property on="SELECT LAB05-2" class="RadioBtnsControl (strict)"("DisabledEnum"=w3323) -> ()  [unwired: 2 in, 2 out]
                n1764 = property on="SELECT LAB05-1" class="RadioBtnsControl (strict)"("DisabledEnum"=w3324) -> ()  [unwired: 2 in, 2 out]
                n1765 = property on="SELECT LAB03-2" class="RadioBtnsControl (strict)"("DisabledEnum"=w3327) -> ()  [unwired: 2 in, 2 out]
                n1766 = property on="SELECT LAB04-1" class="RadioBtnsControl (strict)"("DisabledEnum"=w3326) -> ()  [unwired: 2 in, 2 out]
                n1767 = property on="SELECT LAB04-2" class="RadioBtnsControl (strict)"("DisabledEnum"=w3325) -> ()  [unwired: 2 in, 2 out]
                n1768 = property on="SET LAB05-2" class="Clust (strict)"("DisabledEnum"=w3323) -> ()  [unwired: 2 in, 2 out]
                n1769 = property on="SET LAB05-1" class="Clust (strict)"("DisabledEnum"=w3324) -> ()  [unwired: 2 in, 2 out]
                n1770 = property on="SET LAB03-2" class="Clust (strict)"("DisabledEnum"=w3327) -> ()  [unwired: 2 in, 2 out]
                n1771 = property on="SET LAB04-1" class="Clust (strict)"("DisabledEnum"=w3326) -> ()  [unwired: 2 in, 2 out]
                n1772 = property on="SET LAB04-2" class="Clust (strict)"("DisabledEnum"=w3325) -> ()  [unwired: 2 in, 2 out]
                n1773 = property on="O/I  LAB05-2" class="Bool (strict)"("DisabledEnum"=w3323) -> ()  [unwired: 2 in, 2 out]
                n1774 = property on="O/I  LAB05-1" class="Bool (strict)"("DisabledEnum"=w3324) -> ()  [unwired: 2 in, 2 out]
                n1775 = property on="O/I  LAB04-1" class="Bool (strict)"("DisabledEnum"=w3326) -> ()  [unwired: 2 in, 2 out]
